vi "DPSK调制与解调.vi"() -> ()   [LabVIEW 2013]
uses:
  <vilib>/measure/maspectr.llb/FFT Spectrum (Mag-Phase) for 1 Chan.vi
  <vilib>/Analysis/3filter.llb/Butterworth Filter (DBL).vi
  <vilib>/measure/NI_MAPro.lvlib
  <vilib>/Analysis/NI_AALBase.lvlib
panel:
  out "输出序列（相对码）":u32[](array[numeric])
  out "相对码":i32[](array[numeric]) format="%b"
  in  "标准差":dbl
  out "滤波后波形":dbl[](graph)
  out "2DPSK频谱图":cluster{"f0":dbl, "df":dbl, "magnitude":dbl[]}(graph)
  out "2DPSK信号波形":dbl[](graph)
  out "相对码波形":dbl[](graph)
  out "一个码周期内的点数":dbl
  in  "码速率":dbl
  in  "载频":dbl
  in  "载波相位":dbl
  in  "采样率":dbl
  in  "采样点数":i32
  out "输出序列（绝对码）":u32[](array[numeric])
  in  "输入序列（绝对码）":u32[](array[numeric]) format="%b"
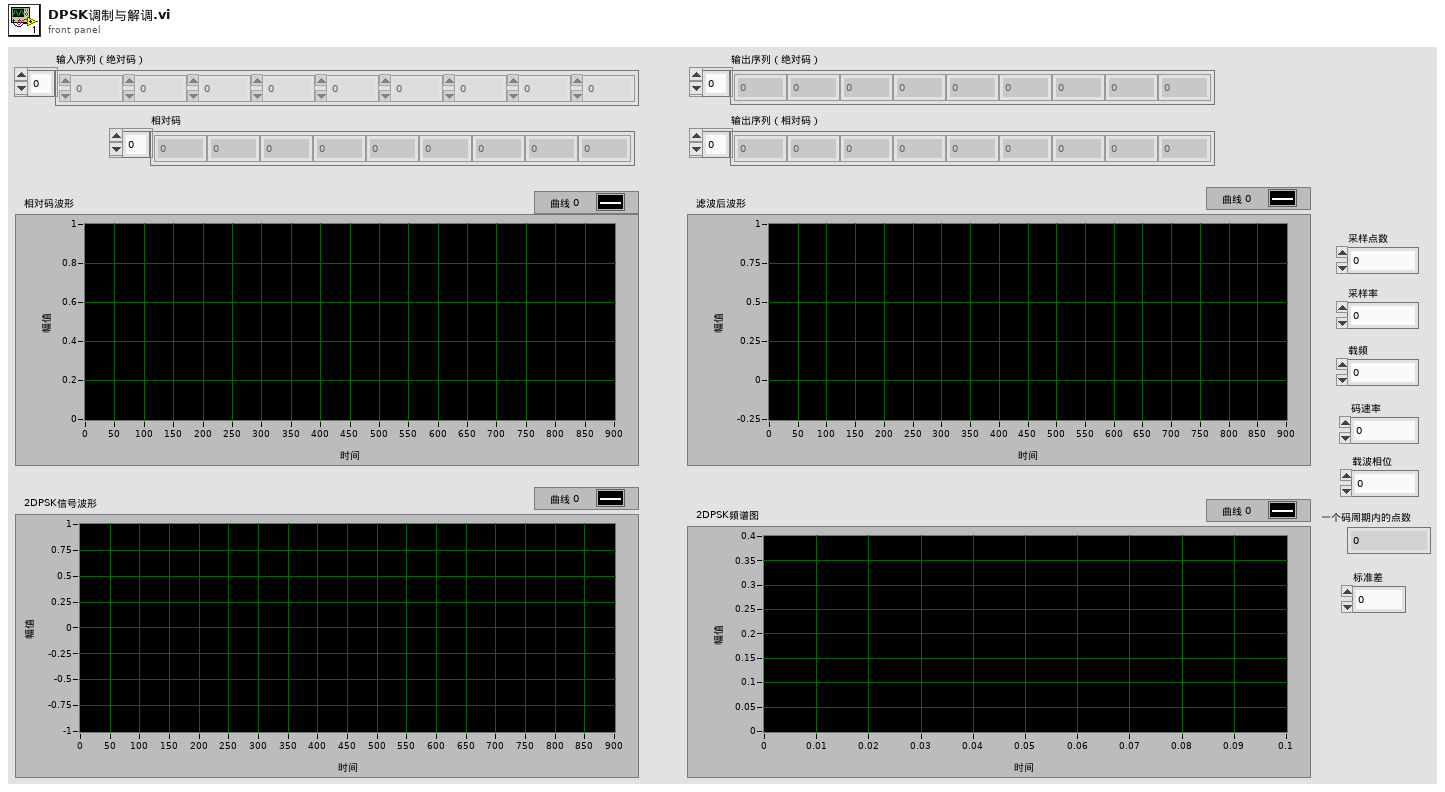
[diagram p1: front panel]
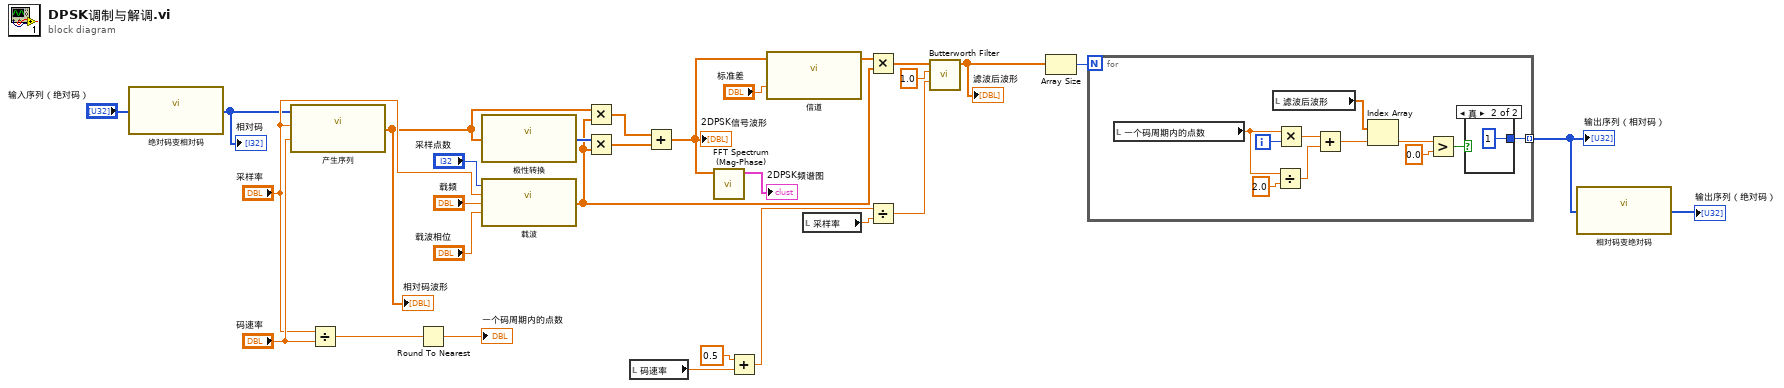
[diagram p0: block diagram]
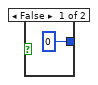
[diagram p2: hidden frame]
diagram:
  n1 = call "绝对码变相对码.vi"("输入信息代码"="输入序列（绝对码）") -> ("相对码"=w3:i32[])
  "相对码" <- w3
  n2 = call "产生序列.vi"("码速率RB"="码速率", "采样率"="采样率", "输入序列"=w3) -> ("输入序列波形"=w19:dbl[])
  "相对码波形" <- w19
  n3 = Divide(x="采样率", y="码速率") -> (x/y=w24:dbl)
  n4 = Round To Nearest(number=w24) -> (nearest integer value=→"一个码周期内的点数":dbl)
  n5 = call "极性转换.vi"("1、0码"=w19) -> ("0、-1码"=w20:i32[])
  n6 = call "载波.vi"("相位输入"="载波相位", "载频"="载频", "采样率"="采样率", "采样点数"="采样点数") -> ("载波信号波形"=w16:dbl[])
  n7 = Multiply(x=w19, y=w16) -> (x*y=w18:dbl[])
  n8 = Multiply(x=w20, y=w16) -> (x*y=w17:dbl[])
  n9 = local read "码速率"() -> (w14:dbl)
  n10 = Add(x=w18, y=w17) -> (x+y=w5:dbl[])
  "2DPSK信号波形" <- w5
  n11 = call-poly <vilib>:"FFT Spectrum (Mag-Phase).vi"("time signal"=w5) -> ("magnitude"=→"2DPSK频谱图":cluster{"f0":dbl, "df":dbl, "magnitude":dbl[]})  [unwired: 6 in, 4 out]
  n12 = Add(x=0.5, y=w14) -> (x+y=w13:dbl)
  n13 = call "信道.vi"("噪声标准差"="标准差", "调制信号"=w5) -> ("信道输出信号"=w4:dbl[])  [unwired: 1 out]
  n14 = local read "采样率"() -> (w12:dbl)
  n15 = Multiply(x=w4, y=w16) -> (x*y=w9:dbl[])
  n16 = Divide(x=w13, y=w12) -> (x/y=w11:dbl)
  n17 = call-poly <vilib>:"Butterworth Filter.vi"("high cutoff freq: fh"=w11, "sampling freq: fs"=1.0, "X"=w9) -> ("Filtered X"=w8:dbl[])  [unwired: 5 in, 1 out]
  "滤波后波形" <- w8
  n18 = Array Size(array=w8) -> (size(s)=w21:i32)
  n19 = for {
    N: w21 -> [_]
    tunnel: [w35] -> w2 mode=indexing
    i -> [w40]
    n20 = local read "一个码周期内的点数"() -> (w37:dbl)
    n21 = local read "滤波后波形"() -> (w32:dbl[])
    n22 = Divide(x=w37, y=2.0) -> (x/y=w38:dbl)
    n23 = Multiply(x=w37, y=w40) -> (x*y=w34:dbl)
    n24 = Add(x=w34, y=w38) -> (x+y=w33:dbl)
    n25 = Index Array(array=w32, index=w33) -> (element=w30:dbl)
    n26 = Greater?(x=w30, y=0.0) -> (0:w36:bool)
    n27 = case shown="真" w36 {
      tunnel: [0 1] -> w35
      frame False {
      }
      frame True {
      }
    }
  }
  "输出序列（相对码）" <- w2
  n28 = call "相对码变绝对码.vi"("相对码"=w2) -> ("绝对码"=→"输出序列（绝对码）":i32[])
